vi "DDS RAM Set.vi"(8 "error in (no error)":errorcluster, 11 "DDS Box Cluster":T8 {"Array of DDS Channels (4)"."Array of DDS Profiles (8)"."Time Step (us)" min=0.0 max=262.14 step=0.004 format="%8.3g"; "Array of DDS Channels (4)"."Channel Parameters"."Ref Clock Rate [MHz]" min=0.0}) -> (0 "error out":errorcluster, 3 "DDS box device reference":T9={"NI USB-8451 device reference"="", "DIO port"=0, "Serial Clock Rate [kHz]"=1000})   [LabVIEW 2015, in "DDS.lvlib"]
uses:
  DDS.lvlib
  Controls/DDS Box Device Reference.ctl
  <vilib>/ni845x/ni845x.llb/ni845xControl.ctl
  Controls/DDS Box Cluster.ctl
  Controls/DDS Channel Array.ctl
  Controls/DDS Channel.ctl
  Controls/DDS Channel Parameters.ctl
  Controls/DDS RAM Destination.ctl
  Controls/DDS Profile Array.ctl
  Controls/DDS Profile.ctl
  Controls/DDS RAM Mode.ctl
  Controls/DDS RAM Timestep.ctl
  Controls/AD9910 registers.ctl
panel:
  out "RAM Set Profile Error":errorcluster[](array[cluster])
  out "start address":u16[](array[numeric])
  out "stop address":u16[](array[numeric])
  out "x-1":u16
  out "DDS Channel":T1={"Power"=FALSE, "Channel Parameters"={"Ref Clock Rate [MHz]"=1000.0, "Full Scale Output\nPower [dBm]"=0.0}, "RAM Enable"=FALSE, "RAM Dest Type"=enum."Frequency", "RAM Default"={"Frequency [MHz]"=0.0, "Amplitude [dBm]"=0.0, "Phase Offset [rad]"=0.0}, "Array of DDS Profiles (8)"=[], "Description"=""} {"Array of DDS Profiles (8)"."Time Step (us)" min=0.0 max=262.14 step=0.004 format="%8.3g"; "Channel Parameters"."Ref Clock Rate [MHz]" min=0.0}
  # "f/f/A"
  # "Mag"
  # "f/f/A"
  # "Mag"
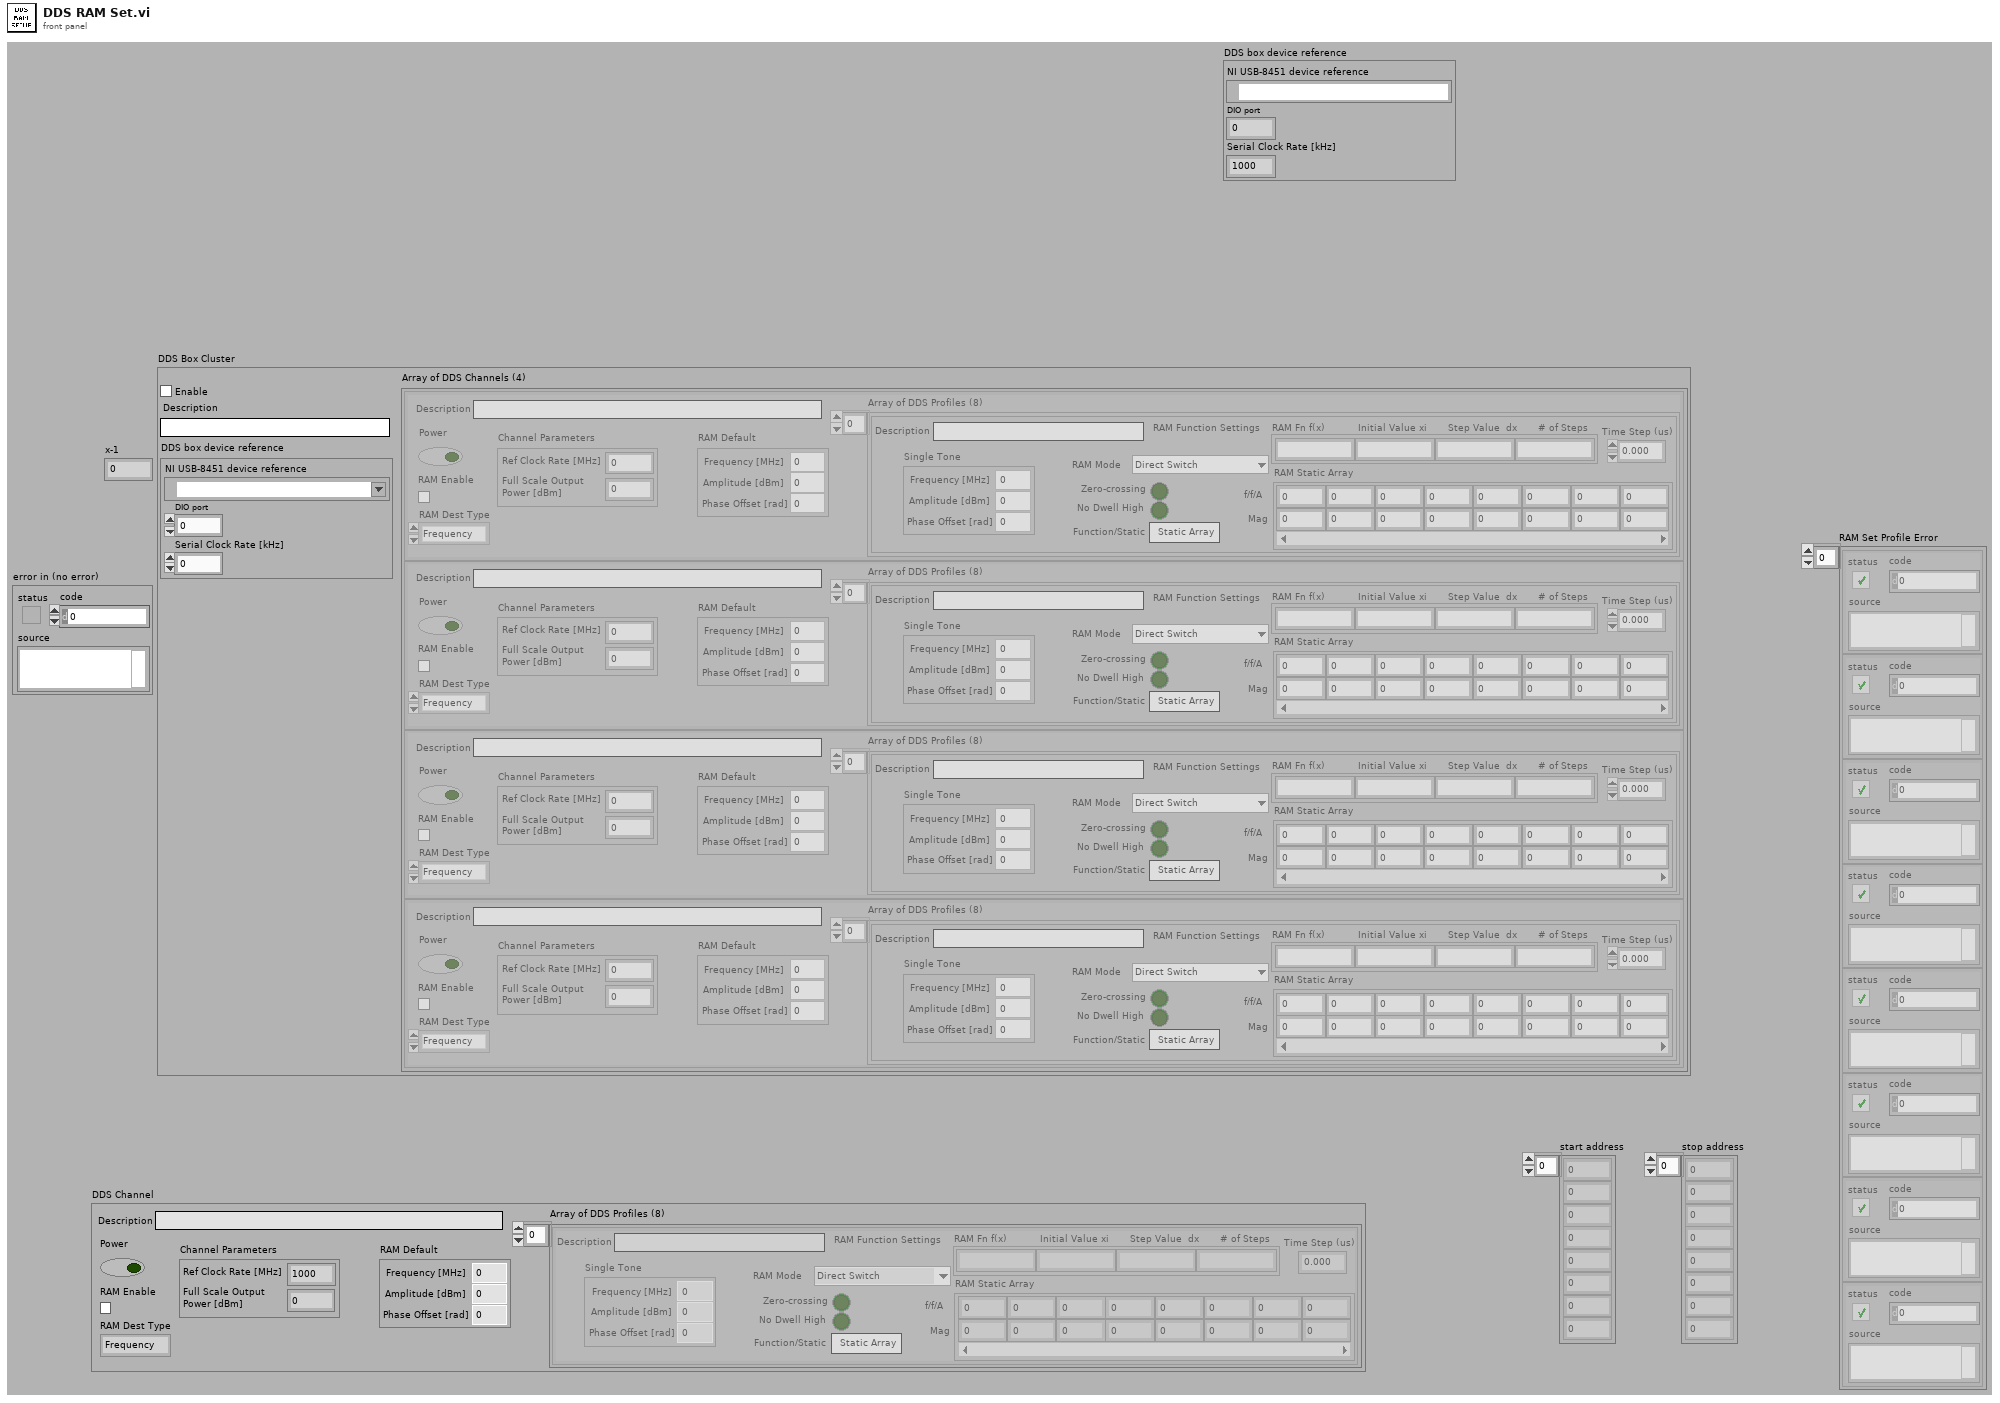
[diagram p1: front panel]
types:
  T1 = typedef "DDS.lvlib/DDS Channel.ctl" = cluster{"Power":bool, "Channel Parameters":T2, "RAM Enable":bool, "RAM Dest Type":T3, "RAM Default":cluster{"Frequency [MHz]":dbl, "Amplitude [dBm]":dbl, "Phase Offset [rad]":dbl}, "Array of DDS Profiles (8)":T4, "Description":string}
  T2 = typedef "DDS.lvlib/DDS Channel Parameters.ctl" = cluster{"Ref Clock Rate [MHz]":dbl, "Full Scale Output\nPower [dBm]":dbl}
  T3 = typedef "DDS.lvlib/DDS RAM Destination.ctl" = enum16{"Frequency", "Phase", "Amplitude", "Polar"}
  T4 = typedef "DDS.lvlib/DDS Profile Array.ctl" = T5[]
  T5 = typedef "DDS.lvlib/DDS Profile.ctl" = cluster{"Single Tone":cluster{"Frequency [MHz]":dbl, "Amplitude [dBm]":dbl, "Phase Offset [rad]":dbl}, "RAM Mode ":T6, "Zero-crossing":bool, "No Dwell High":bool, "Function/Static":bool, "RAM Function Settings":string[], "RAM Static Array":dbl[][], "Description":string, "Time Step (us)":T7}
  T6 = typedef "DDS.lvlib/DDS RAM mode.ctl" = enum16{"Direct Switch", "Ramp Up", "Bidirectional Ramp", "Continuous Bidirectional Ramp", "Continuous Recirculate", "Direct Switch 2", "Direct Switch 3", "Direct Switch 4"}
  T7 = typedef "DDS.lvlib/DDS RAM Timestep.ctl" = dbl
  T8 = typedef "DDS.lvlib/DDS Box Cluster.ctl" = cluster{"DDS box device reference":T9, "Array of DDS Channels (4)":T11, "Enable":bool, "Description":string}
  T9 = typedef "DDS.lvlib/DDS Box Device Reference.ctl" = cluster{"NI USB-8451 device reference":T10, "DIO port":u8, "Serial Clock Rate [kHz]":u16}
  T10 = typedef "ni845xControl.ctl" = refnum<k21>
  T11 = typedef "DDS.lvlib/DDS Channel Array.ctl" = T1[]
  T12 = typedef "DDS.lvlib/DDS RAM Mode.ctl" = enum16{"Direct Switch", "Ramp Up", "Bidirectional Ramp", "Continuous Bidirectional Ramp", "Continuous Recirculate", "Direct Switch 2", "Direct Switch 3", "Direct Switch 4"}
  T13 = cluster{"Frequency [MHz]":dbl, "Amplitude [dBm]":dbl, "Phase Offset [rad]":dbl}
  T14 = typedef "DDS.lvlib/AD9910 registers.ctl" = enum16{"CFR1", "CFR2", "CFR3", "Auxiliary DAC Control", "I/0 Update Rate", "Frequency Tuning Word", "Phase Offset Word", "Amplitude Scale Factor", "Multichip Sync", "Digital Ramp Limit", "Digital Ramp Step Size", "Digital Ramp Rate", "Single Tone Profile 0", "Single Tone Profile 1", "Single Tone Profile 2", "Single Tone Profile 3", "Single Tone Profile 4", "Single Tone Profile 5", "Single Tone Profile 6", "Single Tone Profile 7", "RAM Profile 0", "RAM Profile 1", "RAM Profile 2", "RAM Profile 3", "RAM Profile 4", "RAM Profile 5", "RAM Profile 6", "RAM Profile 7", "RAM"}
  T15 = typedef "DDS.lvlib/DDS RAM Profile.ctl" = cluster{"TimeStep":u16, "Start Address":u16, "Stop Address":u16, "RAM Mode":T12, "No Dwell High":bool, "Zero Crossing":bool}
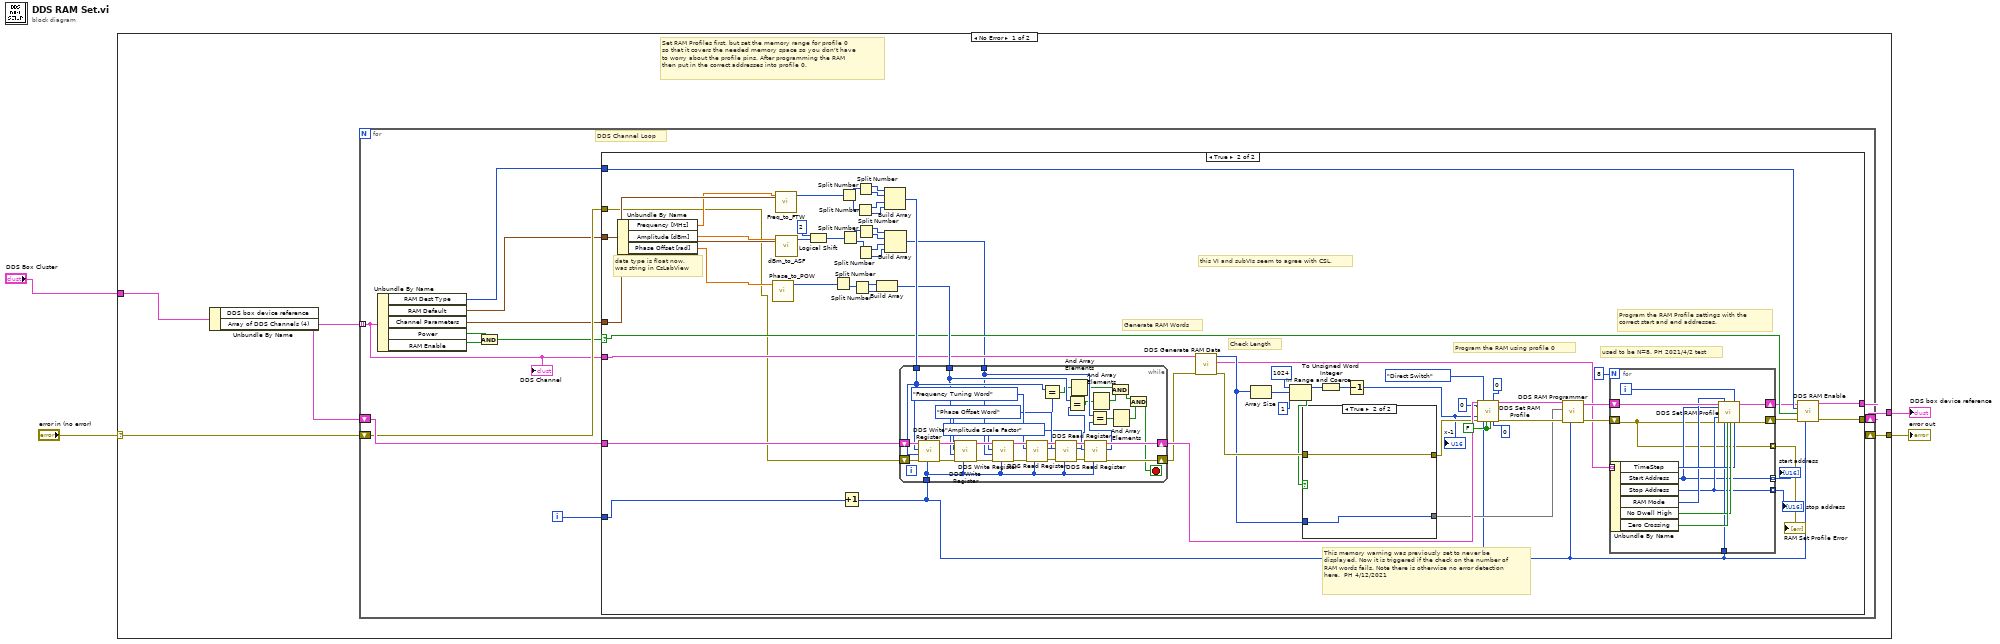
[diagram p0: block diagram]
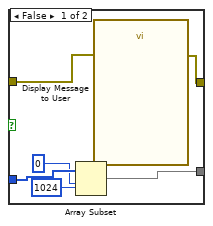
[diagram p3: hidden frame]
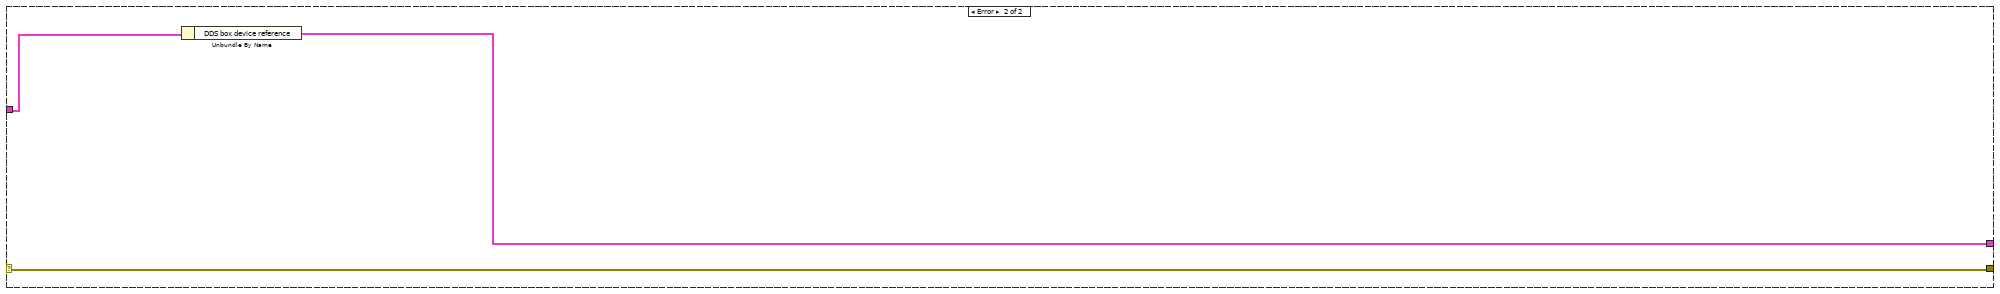
[diagram p4: hidden frame]
diagram:
  n1 = case shown="No Error" "error in (no error)" {
    selector: "error in (no error)" -> [w6 w145]
    tunnel: [w10 w146] -> w4
    tunnel: [w9 w145] -> w3
    tunnel: "DDS Box Cluster" -> [w5 w144]
    frame No Error {
      # "Set RAM Profiles first, but set the memory range for profile 0\nso that it covers the needed memory space so you don't have\nto worry about the profile pins. After programming the RAM\nthen put in the correct addresses into profile 0."
      n2 = Unbundle By Name(w5) -> ("DDS box device reference"=w8:T9, "Array of DDS Channels (4)"=w7:T11)
      n3 = for {
        shift-right: [w22] -> w10
        shift-left: w8 -> [w20]
        shift-right: [w21] -> w9
        shift-left: w6 -> [w19]
        tunnel: w7 -> [w11] mode=indexing
        i -> [w18]
        # "DDS Channel Loop"
        n4 = Unbundle By Name(w11) -> ("RAM Dest Type"=w16:T3, "RAM Default"=w15:T13, "Channel Parameters"=w12:T2, "Power"=w13:bool, "RAM Enable"=w14:bool)
        n5 = And(x=w13, y=w14) -> (x .and. y?=w17:bool)
        n6 = case shown="True" w17 {
          selector: w17 -> [_ w69]
          tunnel: w15 -> [_ w82]
          tunnel: w12 -> [_ w58]
          tunnel: [w24 w71] -> w22
          tunnel: [w23 w70] -> w21
          tunnel: w20 -> [w24 w72]
          tunnel: w19 -> [w23 w29]
          tunnel: w16 -> [_ w68]
          tunnel: w18 -> [_ w61]
          tunnel: w11 -> [_ w60]
          frame False {
          }
          frame True {
            w40 = FALSE ("Zero-crossing")
            # "this VI and subVIs seem to agree with CSL."
            # "data type is float now, \nwas string in CsLabView"
            # "used to be N=8. PH 2021/4/2 test"
            # "This memory warning was previously set to never be displayed. Now it is triggered if the check on the number of RAM words fails. Note there is otherwise no error detection here.  PH 4/12/2021"
            # "Check Length"
            # "Program the RAM Profile settings with the\ncorrect start and end addresses."
            # "Program the RAM using profile 0"
            # "Generate RAM Words"
            n7 = Unbundle By Name(w82) -> ("Frequency [MHz]"=w32:dbl, "Amplitude [dBm]"=w31:dbl, "Phase Offset [rad]"=w30:dbl)
            n8 = call "Phase_to_POW.vi"("Phase (rad.)"=w30) -> ("POW"=w48:u32)  [unwired: 26 in]
            n9 = call "Freq_to_FTW.vi"("Frequency (MHz)"=w32, "Channel Parameters"=w58) -> ("FTW (32bit)"=w59:u32)  [unwired: 25 in]
            n10 = call "dBm_to_ASF.vi"("Amplitude (dBm)"=w31, "Channel Parameters"=w58) -> ("ASF"=w51:u32)  [unwired: 25 in]
            n11 = Logical Shift(y=i8 2, x=w51) -> (x << y=w50:u32)
            n12 = Split Number(x=w48) -> (lo(x)=w49:u16)  [unwired: 1 out]
            n13 = Split Number(x=w59) -> (hi(x)=w89:u16, lo(x)=w90:u16)
            n14 = Split Number(x=w50) -> (hi(x)=w53:u16, lo(x)=w52:u16)
            n15 = Increment(x=w61) -> (x+1=w36:i32)
            n16 = Split Number(x=w49) -> (hi(x)=w84:u8, lo(x)=w83:u8)
            n17 = Split Number(x=w90) -> (hi(x)=w86:u8, lo(x)=w85:u8)
            n18 = Split Number(x=w89) -> (hi(x)=w88:u8, lo(x)=w87:u8)
            n19 = Split Number(x=w52) -> (hi(x)=w56:u8, lo(x)=w57:u8)
            n20 = Split Number(x=w53) -> (hi(x)=w54:u8, lo(x)=w55:u8)
            n21 = Build Array(w84, w83) -> (w80:u8[])
            n22 = Build Array(w88, w87, w86, w85) -> (w81:u8[])
            n23 = Build Array(w54, w55, w56, w57) -> (w47:u8[])
            n24 = while {
              tunnel: w81 -> [w124]
              tunnel: w47 -> [w122]
              tunnel: w80 -> [w123]
              tunnel: w36 -> [w126]
              shift-right: [w130] -> w79
              shift-left: w72 -> [w139]
              shift-right: [w131] -> w78
              shift-left: w29 -> [w138]
              stop <- w112 stop-if-true
              w127 = AD9910_registers."Amplitude Scale Factor" ("Register")
              w128 = AD9910_registers."Phase Offset Word" ("Register")
              w129 = AD9910_registers."Frequency Tuning Word" ("Register")
              n25 = call "DDS Write Register.vi"("channel number (1)"=w126, "error in (no error)"=w138, "Write Data"=w124, "Register"=w129, "DDS ref in"=w139) -> ("error out"=w142:errorcluster, "DDS ref out"=w143:T9)  [unwired: 4 in, 1 out]
              n26 = call "DDS Write Register.vi"("channel number (1)"=w126, "error in (no error)"=w142, "Write Data"=w123, "Register"=w128, "DDS ref in"=w143) -> ("error out"=w140:errorcluster, "DDS ref out"=w141:T9)  [unwired: 4 in, 1 out]
              n27 = call "DDS Write Register.vi"("channel number (1)"=w126, "error in (no error)"=w140, "Write Data"=w122, "Register"=w127, "DDS ref in"=w141) -> ("error out"=w134:errorcluster, "DDS ref out"=w137:T9)  [unwired: 4 in, 1 out]
              n28 = call "DDS Read Register.vi"("channel number (1)"=w126, "error in (no error)"=w134, "Register"=w129, "DDS ref in"=w137) -> ("error out"=w133:errorcluster, "Read data"=w125:u8[], "DDS ref out"=w136:T9)  [unwired: 5 in]
              n29 = Equal?(x=w124, y=w125) -> (x = y?=w119:bool[])
              n30 = call "DDS Read Register.vi"("channel number (1)"=w126, "error in (no error)"=w133, "Register"=w128, "DDS ref in"=w136) -> ("error out"=w132:errorcluster, "Read data"=w121:u8[], "DDS ref out"=w135:T9)  [unwired: 5 in]
              n31 = Equal?(x=w123, y=w121) -> (x = y?=w117:bool[])
              n32 = And Array Elements(Boolean array=w119) -> (logical AND=w115:bool)
              n33 = call "DDS Read Register.vi"("channel number (1)"=w126, "error in (no error)"=w132, "Register"=w127, "DDS ref in"=w135) -> ("error out"=w131:errorcluster, "Read data"=w120:u8[], "DDS ref out"=w130:T9)  [unwired: 5 in]
              n34 = Equal?(x=w122, y=w120) -> (x = y?=w118:bool[])
              n35 = And Array Elements(Boolean array=w117) -> (logical AND=w116:bool)
              n36 = And(x=w115, y=w116) -> (x .and. y?=w113:bool)
              n37 = And Array Elements(Boolean array=w118) -> (logical AND=w114:bool)
              n38 = And(x=w113, y=w114) -> (x .and. y?=w112:bool)
            }
            n39 = call "DDS Generate RAM Data.vi"("error in (no error)"=w78, "DDS Channel"=w60) -> ("error out"=w63:errorcluster, "RAM Profile Array"=w37:T15[], "RAM Word Array"=w42:u32[])  [unwired: 7 in]
            n40 = Array Size(array=w42) -> (size(s)=w64:i32)
            n41 = In Range and Coerce(upper limit=1024, x=w64, lower limit=1) -> (coerced(x)=w46:i32, In Range?=w25:bool)
            n42 = case shown="True" w25 {
              tunnel: w63 -> [w109 w111]
              tunnel: [w108 w111] -> w62
              tunnel: w42 -> [w107 w110]
              tunnel: [w105 w110] -> w41
              frame False {
                n43 = Array Subset(array=w107, index=0, length=1024) -> (w105:u32[])
                n44 = call "Display Message to User"("error in (no error)"=w109) -> ("error out"=w108:errorcluster)  [unwired: 9 in, 1 out]
              }
              frame True {
              }
            }
            n45 = To Unsigned Word Integer(number=w46) -> (unsigned 16bit integer=w45:u16)
            n46 = Decrement(x=w45) -> (x-1=w44:u16)
            "x-1" <- w44
            n47 = call "DDS Set RAM Profile.vi"("DDS ref in"=w79, "Start Address"=u16 0, "End Address"=w44, "error in (no error)"=w62, "RAM mode"=DDS_RAM_Mode."Direct Switch", "channel number (1)"=w36, "Zero-crossing"=w40, "No Dwell High"=w40, "Profile (0)"=u8 0, "Step Rate"=u16 0) -> ("DDS ref out"=w75:T9, "error out"=w74:errorcluster)  [unwired: 7 in, 1 out]
            n48 = call "DDS RAM Programmer.vi"("channel number (1)"=w36, "error in (no error)"=w74, "RAM Word Array"=w41, "DDS ref in"=w75) -> ("error out"=w38:errorcluster, "DDS ref out"=w39:T9)  [unwired: 6 in]
            n49 = for {
              N: 8 -> [_]
              shift-right: [w101] -> w34
              shift-left: w39 -> [w103]
              shift-right: [w100] -> w33
              shift-left: w38 -> [w91]
              tunnel: w37 -> [w99] mode=indexing
              tunnel: w36 -> [w95]
              tunnel: [w93] -> w28 mode=indexing
              tunnel: [w92] -> w27 mode=indexing
              tunnel: [w91] -> w26 mode=indexing
              i -> [w102]
              n50 = Unbundle By Name(w99) -> ("TimeStep"=w96:u16, "Start Address"=w92:u16, "Stop Address"=w93:u16, "RAM Mode"=w94:T12, "No Dwell High"=w97:bool, "Zero Crossing"=w98:bool)
              n51 = call "DDS Set RAM Profile.vi"("DDS ref in"=w103, "Start Address"=w92, "End Address"=w93, "error in (no error)"=w91, "RAM mode"=w94, "channel number (1)"=w95, "Zero-crossing"=w98, "No Dwell High"=w97, "Profile (0)"=w102, "Step Rate"=w96) -> ("DDS ref out"=w101:T9, "error out"=w100:errorcluster)  [unwired: 7 in, 1 out]
            }
            "stop address" <- w28
            "start address" <- w27
            "RAM Set Profile Error" <- w26
            n52 = call "DDS RAM Enable.vi"("channel number (1)"=w36, "error in"=w33, "RAM Enable"=w69, "RAM Dest Type"=w68, "DDS ref in"=w34) -> ("error out"=w70:errorcluster, "DDS ref out"=w71:T9)  [unwired: 5 in]
          }
        }
        "DDS Channel" <- w11
      }
    }
    frame Error {
      n53 = Unbundle By Name(w144) -> ("DDS box device reference"=w146:T9)
    }
  }
  "error out" <- w3
  "DDS box device reference" <- w4
